vi "Tester.vi"() -> ()   [LabVIEW 2019, in "Simple Queue Message.lvlib"]
uses:
  Simple Queue Message.lvlib
panel:
  out "state":string
  out "payload":string
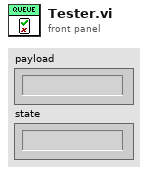
[diagram p1: front panel]
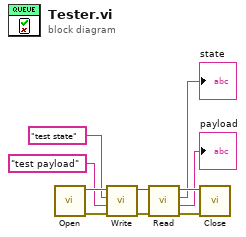
[diagram p0: block diagram]
diagram:
  n1 = call "Open.vi"() -> ("error out"=w5:errorcluster, "queue out"=w10:refnum<queue>)  [unwired: 10 in]
  n2 = call "Write.vi"("error in (no error)"=w5, "payload"="test payload", "state"="test state", "queue"=w10) -> ("error out"=w4:errorcluster, "queue out"=w7:refnum<queue>)  [unwired: 6 in]
  n3 = call "Read.vi"("error in (no error)"=w4, "queue"=w7) -> ("error out"=w3:errorcluster, "payload"=→"payload":string, "state"=→"state":string, "queue out"=w6:refnum<queue>)  [unwired: 6 in]
  n4 = call "Close.vi"("error in (no error)"=w3, "queue out"=w6) -> ()  [unwired: 9 in, 1 out]
